vi "GL InitPID.vi"(6 "error in":errorcluster, 7 "ControPrams":cluster{"KD":i32, "KI":dbl, "KP":i32, "IL":i32}, 8 "Axis":T1 items=["Axis 1", "Axis 2", "Axis 3", "Axis 4", "Axis 5", "Axis 6", "Axis 7", "Axis 8"], 9 "Galil.IGalil":refnum<k7>) -> (0 "error out":errorcluster, 2 "Axis Out Output":T1 items=["Axis 1", "Axis 2", "Axis 3", "Axis 4", "Axis 5", "Axis 6", "Axis 7", "Axis 8"], 3 "ref out":refnum<k7>)   [LabVIEW 2022 SP3]
doc: "Sets the operation mode for an axis or vector space."
uses:
  GL Axis Control.ctl
  Command Menu.ctl
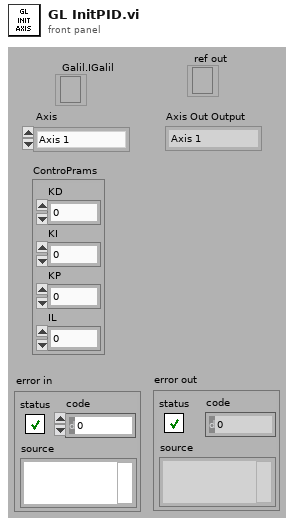
[diagram p1: front panel]
types:
  T1 = typedef "GL Axis Control.ctl" = u16
  T2 = typedef "Command Menu.ctl" = enum16{"CommandPassThrough", "Abort Motion", "Define Pos", "Velocity", "Acceleration", "Deceleration", "Position Rel", "Postion Abs", "Begin Move", "After Move", "Home", "KI", "KD", "KP", "IL", "Config I/O", "Set Bit", "Clear Bit", "Motor Off", "Moto On", "Status", "Execute", "Halt Execute", "HX Status", "Tell Velocity", "Check Motion", "BreakPoint", "Tell Position", "Current Code Line", "Tell Switches", "OC Force On", "OC Off", "Pos Soft Limit", "Rev Soft Limit"}
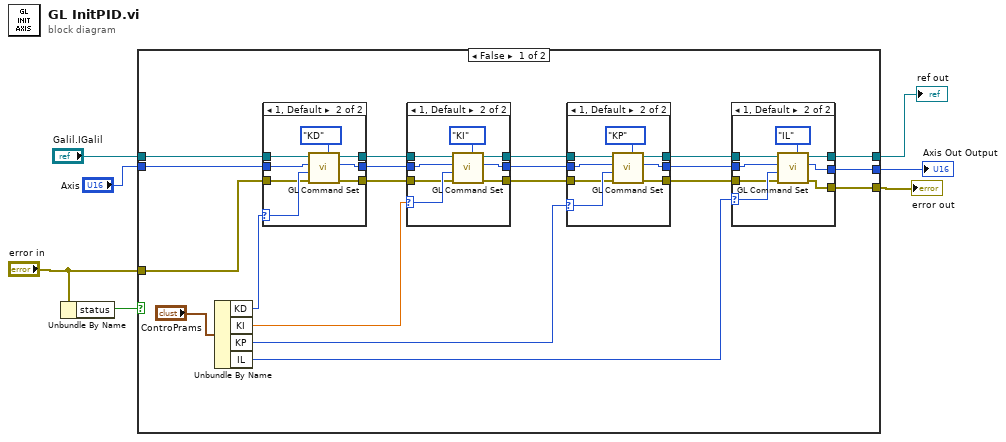
[diagram p0: block diagram]
diagram:
  n1 = Unbundle By Name("error in") -> ("status"=w5:bool)
  n2 = case shown="False" w5 {
    tunnel: "error in" -> [w18 w74]
    tunnel: [w17 w74] -> w6
    tunnel: [w16 w73] -> w4
    tunnel: "Galil.IGalil" -> [w15 w72]
    tunnel: "Axis" -> [w14 w73]
    tunnel: [w8 w72] -> w1
    frame False {
      n3 = Unbundle By Name("ControPrams") -> ("KD"=w12:i32, "KI"=w11:dbl, "KP"=w10:i32, "IL"=w9:i32)
      n4 = case shown="1, Default" w12 {
        selector: w12 -> [_ w37]
        tunnel: [w30 w36] -> w27
        tunnel: w15 -> [w30 w35]
        tunnel: w14 -> [w29 w34]
        tunnel: [w29 w33] -> w24
        tunnel: [w28 w32] -> w19
        tunnel: w18 -> [w28 w31]
        frame 0 {
        }
        frame 1, Default {
          n5 = call "GL Command Set.vi"("Command"=Command_Menu."KD", "error in (no error)"=w31, "Value"=w37, "Axis"=w34, "Galil.IGalil"=w35) -> ("error out"=w32:errorcluster, "Axis Out"=w33:T1, "ref out"=w36:refnum<k7>)  [unwired: 2 in, 2 out]
        }
      }
      n6 = case shown="1, Default" w11 {
        selector: w11 -> [_ w48]
        tunnel: [w41 w47] -> w26
        tunnel: w27 -> [w41 w46]
        tunnel: w24 -> [w40 w45]
        tunnel: [w40 w42] -> w23
        tunnel: [w39 w44] -> w20
        tunnel: w19 -> [w39 w43]
        frame 0 {
        }
        frame 1, Default {
          n7 = call "GL Command Set.vi"("Command"=Command_Menu."KI", "error in (no error)"=w43, "Value"=w48, "Axis"=w45, "Galil.IGalil"=w46) -> ("error out"=w44:errorcluster, "Axis Out"=w42:T1, "ref out"=w47:refnum<k7>)  [unwired: 2 in, 2 out]
        }
      }
      n8 = case shown="1, Default" w10 {
        selector: w10 -> [_ w59]
        tunnel: [w52 w58] -> w25
        tunnel: w26 -> [w52 w57]
        tunnel: w23 -> [w51 w56]
        tunnel: [w51 w55] -> w22
        tunnel: [w50 w54] -> w21
        tunnel: w20 -> [w50 w53]
        frame 0 {
        }
        frame 1, Default {
          n9 = call "GL Command Set.vi"("Command"=Command_Menu."KP", "error in (no error)"=w53, "Value"=w59, "Axis"=w56, "Galil.IGalil"=w57) -> ("error out"=w54:errorcluster, "Axis Out"=w55:T1, "ref out"=w58:refnum<k7>)  [unwired: 2 in, 2 out]
        }
      }
      n10 = case shown="1, Default" w9 {
        selector: w9 -> [_ w70]
        tunnel: [w62 w69] -> w8
        tunnel: w25 -> [w62 w68]
        tunnel: w22 -> [w61 w67]
        tunnel: w21 -> [w63 w66]
        tunnel: [w63 w65] -> w17
        tunnel: [w61 w64] -> w16
        frame 0 {
        }
        frame 1, Default {
          n11 = call "GL Command Set.vi"("Command"=Command_Menu."IL", "error in (no error)"=w66, "Value"=w70, "Axis"=w67, "Galil.IGalil"=w68) -> ("error out"=w65:errorcluster, "Axis Out"=w64:T1, "ref out"=w69:refnum<k7>)  [unwired: 2 in, 2 out]
        }
      }
    }
    frame True {
    }
  }
  "error out" <- w6
  "ref out" <- w1
  "Axis Out Output" <- w4
